vi "crio1_fpga.vi"() -> ()   [LabVIEW 2012]
uses:
  <vilib>/LabVIEW Targets/FPGA/cRIO/shared/nicrio_ModuleControls/nicrio_cRIO-9871_BaudRateEnum.ctl
  <vilib>/LabVIEW Targets/FPGA/cRIO/shared/nicrio_ModuleControls/nicrio_cRIO-9871_DataBitsEnum.ctl
  <vilib>/LabVIEW Targets/FPGA/cRIO/shared/nicrio_ModuleControls/nicrio_cRIO-9871_ParityEnum.ctl
  <vilib>/LabVIEW Targets/FPGA/cRIO/shared/nicrio_ModuleControls/nicrio_cRIO-9871_StopBitsEnum.ctl
  <vilib>/rvi/eio/common/nirviEmuTemplateMethod_errors.vi
  <vilib>/rvi/eio/common/nirviEmuTemplatePropertySet_noerrors.vi
  <vilib>/eio/EIONode/EIONode.xnode
  <vilib>/eio/EIOMethodNode/EIOMethodNode.xnode
  <vilib>/eio/EIOPropertyNode/EIOPropertyNode.xnode
  <vilib>/rvi/eio/common/nirviEmuTemplatePropertyGet_errors.vi
  <vilib>/rvi/eio/common/nirviEmuTemplatePropertyGet_noerrors.vi
  <vilib>/rvi/eio/common/nirviEmuTemplatePropertySet_errors.vi
panel:
  out "interlocked tripped":bool
  out "DI Gate Valves":bool[](array[boolean])
  in  "Mod8/CH2":bool
  in  "Mod8/CH4":bool
  in  "Mod8/CH3":bool
  out "DIO OUTPUT":bool[](array[boolean])
  out "Convectron 2":u8[](array[numeric])
  out "Ion gauge 1":u8[](array[numeric])
  out "Convectron 1":u8[](array[numeric])
  out "Ion gauge 2":u8[](array[numeric])
  in  "R45 Switch magnet Aperture":bool
  in  "R45 Switch magnet faraday cup":bool
  out "Analog input":fxp<+/-,26,5>[](array[numeric]) format="%.23g"
  in  "Analog Output":fxp<+/-,26,5>[](array[numeric])=[0.0, 0.0, 0.0, 0.0, 0.0, 0.0, 0.0, 0.0] format="%.23g"
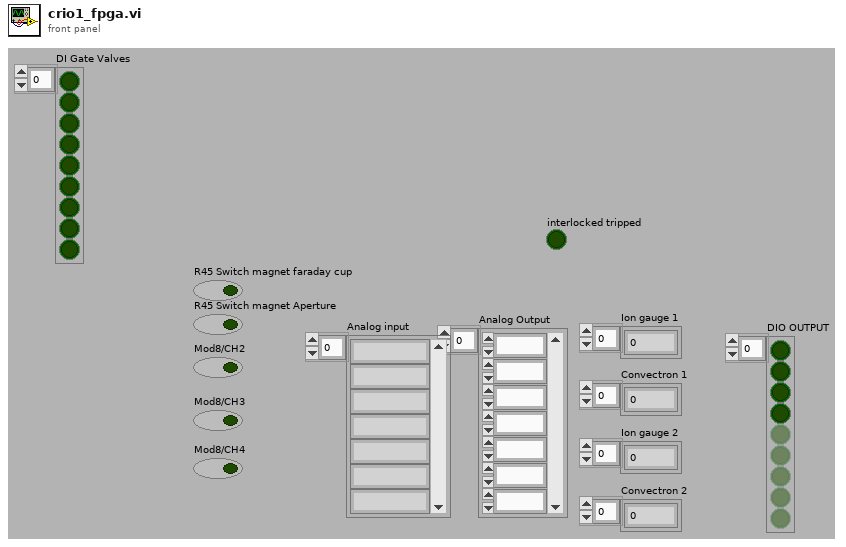
[diagram p1: front panel]
types:
  T1 = typedef "nicrio_cRIO-9871_StopBitsEnum.ctl" = enum8{"1", "1.5", "2"}
  T2 = typedef "nicrio_cRIO-9871_ParityEnum.ctl" = enum8{"None", "Odd", "Even", "Mark", "Space"}
  T3 = typedef "nicrio_cRIO-9871_DataBitsEnum.ctl" = enum8{"5", "6", "7", "8"}
  T4 = typedef "nicrio_cRIO-9871_BaudRateEnum.ctl" = enum16{"75 bps", "110 bps", "134 bps", "150 bps", "300 bps", "600 bps", "1200 bps", "1800 bps", "2400 bps", "4800 bps", "7200 bps", "9600 bps", "14.4 kbps", "19.2 kbps", "28.8 kbps", "38.4 kbps", "57.6 kbps", "115.2 kbps", "230.4 kbps", "460.8 kbps", "921.6 kbps"}
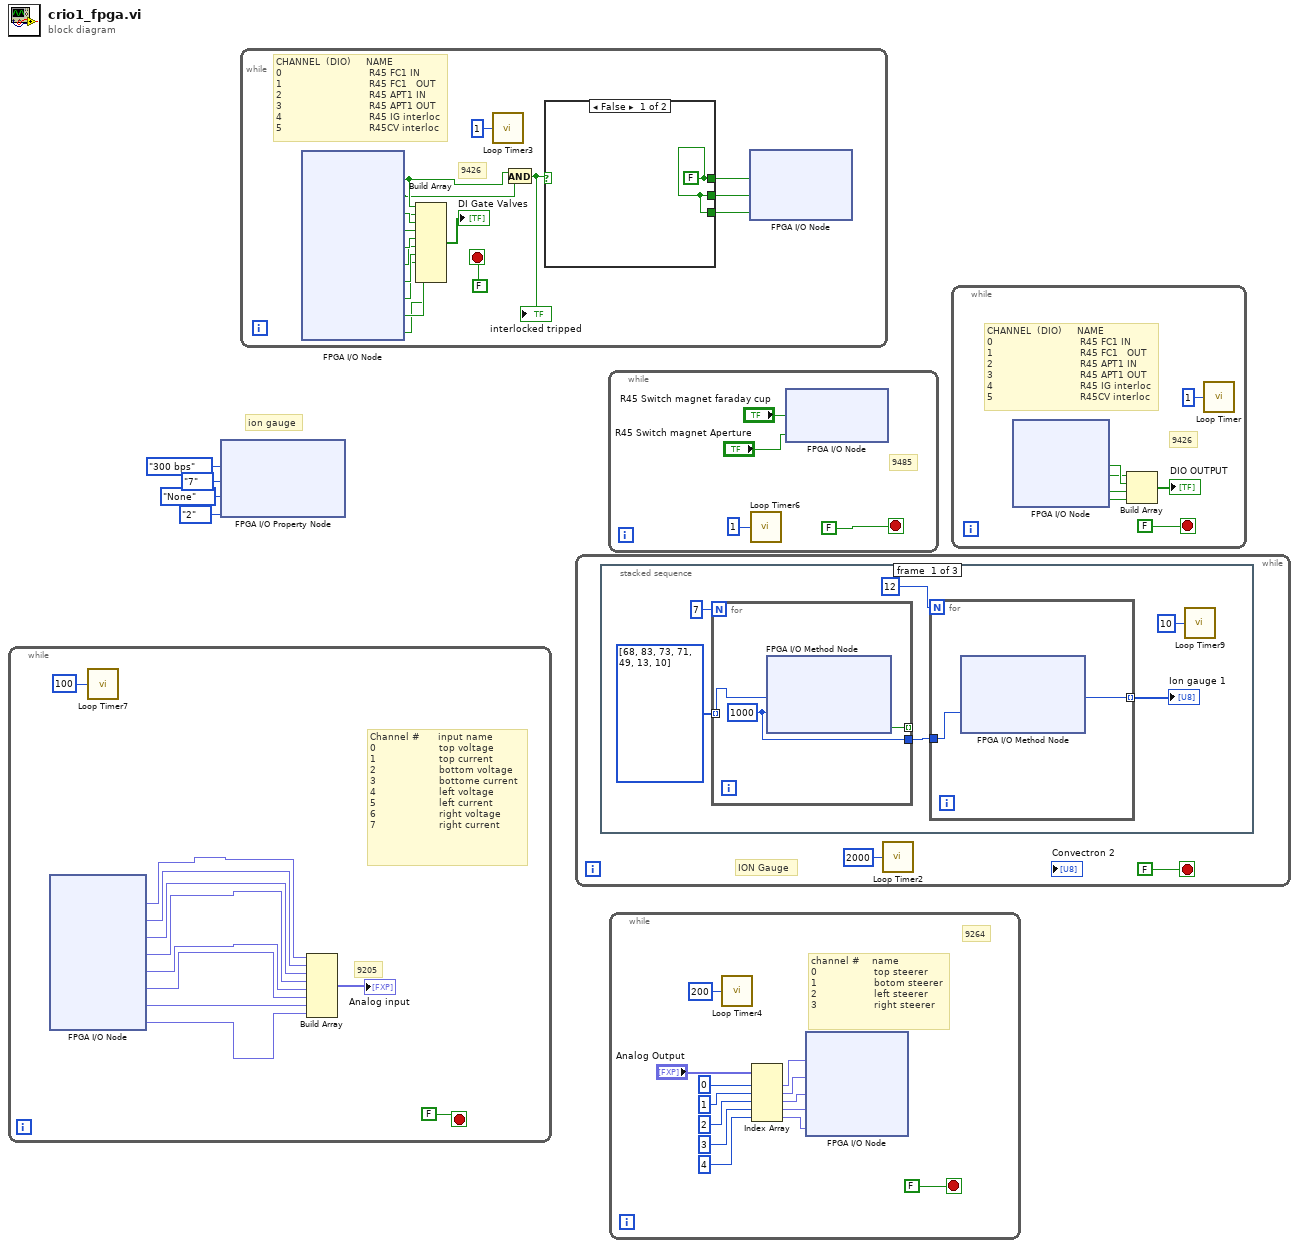
[diagram p0: block diagram]
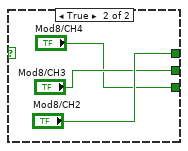
[diagram p2: hidden frame]
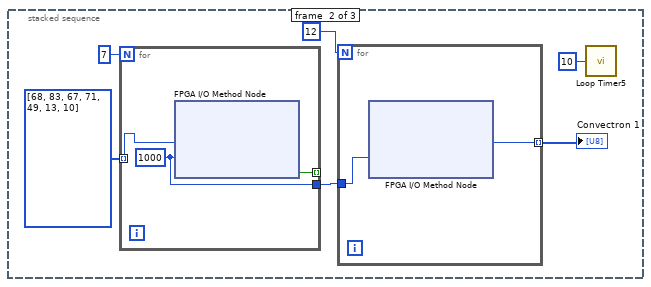
[diagram p3: hidden frame]
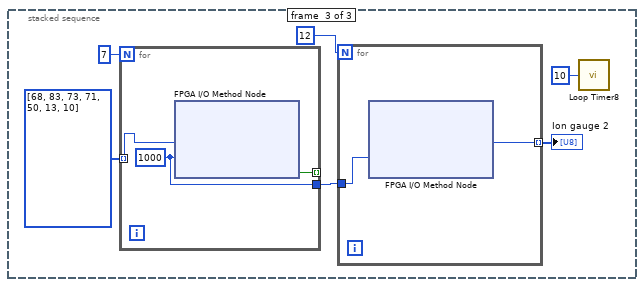
[diagram p4: hidden frame]
diagram:
  # "ion gauge"
  n1 = while {
    stop <- FALSE stop-if-true
    # "Channel #      input name\n0                     top voltage\n1                     top current\n2                     bottom voltage\n3                     bottome current\n4                     left voltage\n5                     left current\n6                     right voltage\n7                     right current"
    # "9205"
    n2 = xnode "FPGA I/O Node"() -> ("Mod1/AI0"=w13:fxp<+/-,26,5>, "Mod1/AI1"=w12:fxp<+/-,26,5>, "Mod1/AI2"=w11:fxp<+/-,26,5>, "Mod1/AI3"=w10:fxp<+/-,26,5>, "Mod1/AI4"=w9:fxp<+/-,26,5>, "Mod1/AI5"=w8:fxp<+/-,26,5>, "Mod1/AI6"=w7:fxp<+/-,26,5>, "Mod1/AI7"=w6:fxp<+/-,26,5>)  [unwired: 8 in, 8 out]
    n3 = call "Loop Timer7"("Count(mSec)"=u32 100 ("Count(Ticks)")) -> ()  [unwired: 1 out]
    n4 = Build Array(w13, w12, w11, w10, w9, w8, w7, w6) -> (→"Analog input":fxp<+/-,26,5>[])
  }
  n5 = xnode "FPGA I/O Property Node"("Baud Rate"=nicrio_cRIO-9871_BaudRateEnum."300 bps", "Data Bits"=nicrio_cRIO-9871_DataBitsEnum."7", "Parity"=nicrio_cRIO-9871_ParityEnum."None", "Stop Bits"=nicrio_cRIO-9871_StopBitsEnum."2") -> ()  [unwired: 1 in, 1 out]
  n6 = while {
    stop <- FALSE stop-if-true
    # "9426"
    # "CHANNEL  (DIO)     NAME\n0                             R45 FC1 IN\n1                             R45 FC1   OUT\n2                             R45 APT1 IN\n3                             R45 APT1 OUT\n4                             R45 IG interloc\n5                             R45CV interloc"
    n7 = xnode "FPGA I/O Node"() -> ("Mod7/DI4"=w21:bool, "Mod7/DI5"=w20:bool, "Mod7/DI6"=w29:bool, "Mod7/DI7"=w28:bool, "Mod7/DI8"=w27:bool, "Mod7/DI9"=w26:bool, "Mod7/DI10"=w19:bool, "Mod7/DI11"=w18:bool, "Mod7/DI12"=w17:bool, "Mod7/DI13"=w16:bool)  [unwired: 10 in, 10 out]
    n8 = Build Array(w21, w20, w29, w28, w27, w26, w19, w18, w17, w16) -> (→"DI Gate Valves":bool[])
    n9 = call "Loop Timer3"("Count(uSec)"=u32 1 ("Count(Ticks)")) -> ()  [unwired: 1 out]
    n10 = And(x=w21, y=w20) -> (x .and. y?=w22:bool)
    "interlocked tripped" <- w22
    n11 = case shown="False" w22 {
      tunnel: [w33 "Mod8/CH2"] -> w25
      tunnel: [w33 "Mod8/CH3"] -> w24
      tunnel: [w33 "Mod8/CH4"] -> w23
      frame False {
        w33 = FALSE ("Mod8/CH2")
      }
      frame True {
      }
    }
    n12 = xnode "FPGA I/O Node"("Mod8/CH2"=w25, "Mod8/CH3"=w24, "Mod8/CH4"=w23) -> ()  [unwired: 3 in, 3 out]
  }
  n13 = while {
    stop <- FALSE stop-if-true
    # "ION Gauge"
    n14 = stacked-sequence {
      frame #0 {
        n15 = for {
          N: 7 -> [_]
          tunnel: [w49] -> w44
          tunnel: [w48] -> _ mode=indexing
          tunnel: u8[] [68, 83, 73, 71, 49, 13, 10] ("unsigned byte array") -> [w47] mode=indexing
          w49 = 1000 ("Timeout (ms)")
          n16 = xnode "FPGA I/O Method Node"("Data"=w47, "Timeout (ms)"=w49) -> ("Timed Out"=w48:bool)  [unwired: 1 in, 1 out]
        }
        n17 = for {
          N: 12 -> [_]
          tunnel: w44 -> [w46]
          tunnel: [w45] -> w40 mode=indexing
          n18 = xnode "FPGA I/O Method Node"("Timeout (ms)"=w46) -> ("Data"=w45:u8)  [unwired: 1 in, 2 out]
        }
        "Ion gauge 1" <- w40
        n19 = call "Loop Timer9"("Count(mSec)"=u32 10 ("Count(Ticks)")) -> ()  [unwired: 1 out]
      }
      frame #1 {
        n20 = for {
          N: 7 -> [_]
          tunnel: [w60] -> w55
          tunnel: [w59] -> _ mode=indexing
          tunnel: u8[] [68, 83, 67, 71, 49, 13, 10] ("unsigned byte array") -> [w58] mode=indexing
          w60 = 1000 ("Timeout (ms)")
          n21 = xnode "FPGA I/O Method Node"("Data"=w58, "Timeout (ms)"=w60) -> ("Timed Out"=w59:bool)  [unwired: 1 in, 1 out]
        }
        n22 = for {
          N: 12 -> [_]
          tunnel: w55 -> [w57]
          tunnel: [w56] -> w51 mode=indexing
          n23 = xnode "FPGA I/O Method Node"("Timeout (ms)"=w57) -> ("Data"=w56:u8)  [unwired: 1 in, 2 out]
        }
        "Convectron 1" <- w51
        n24 = call "Loop Timer5"("Count(mSec)"=u32 10 ("Count(Ticks)")) -> ()  [unwired: 1 out]
      }
      frame #2 {
        n25 = for {
          N: 7 -> [_]
          tunnel: [w71] -> w66
          tunnel: [w70] -> _ mode=indexing
          tunnel: u8[] [68, 83, 73, 71, 50, 13, 10] ("unsigned byte array") -> [w69] mode=indexing
          w71 = 1000 ("Timeout (ms)")
          n26 = xnode "FPGA I/O Method Node"("Data"=w69, "Timeout (ms)"=w71) -> ("Timed Out"=w70:bool)  [unwired: 1 in, 1 out]
        }
        n27 = for {
          N: 12 -> [_]
          tunnel: w66 -> [w68]
          tunnel: [w67] -> w62 mode=indexing
          n28 = xnode "FPGA I/O Method Node"("Timeout (ms)"=w68) -> ("Data"=w67:u8)  [unwired: 1 in, 2 out]
        }
        "Ion gauge 2" <- w62
        n29 = call "Loop Timer8"("Count(mSec)"=u32 10 ("Count(Ticks)")) -> ()  [unwired: 1 out]
      }
    }
    n30 = call "Loop Timer2"("Count(mSec)"=u32 2000 ("Count(Ticks)")) -> ()  [unwired: 1 out]
  }
  n31 = while {
    stop <- FALSE stop-if-true
    # "9485"
    n32 = call "Loop Timer6"("Count(mSec)"=u32 1 ("Count(Ticks)")) -> ()  [unwired: 1 out]
    n33 = xnode "FPGA I/O Node"("Mod8/CH0"="R45 Switch magnet faraday cup", "Mod8/CH1"="R45 Switch magnet Aperture") -> ()  [unwired: 2 in, 2 out]
  }
  n34 = while {
    stop <- FALSE stop-if-true
    # "9264"
    # "channel #    name\n0                   top steerer\n1                   botom steerer\n2                   left steerer\n3                   right steerer"
    n35 = call "Loop Timer4"("Count(mSec)"=u32 200 ("Count(Ticks)")) -> ()  [unwired: 1 out]
    n36 = Index Array(array="Analog Output", index #1=0 ("index"), index #2=1 ("index"), index #3=2 ("index"), index #4=3 ("index"), index #5=4 ("index")) -> (element #1=w81:fxp<+/-,26,5>, element #2=w80:fxp<+/-,26,5>, element #3=w79:fxp<+/-,26,5>, element #4=w78:fxp<+/-,26,5>, element #5=w76:fxp<+/-,26,5>)
    n37 = xnode "FPGA I/O Node"("Mod2/AO0"=w81, "Mod2/AO1"=w80, "Mod2/AO2"=w79, "Mod2/AO3"=w78, "Mod2/AO4"=w76) -> ()  [unwired: 5 in, 5 out]
  }
  n38 = while {
    stop <- FALSE stop-if-true
    # "9426"
    # "CHANNEL  (DIO)     NAME\n0                             R45 FC1 IN\n1                             R45 FC1   OUT\n2                             R45 APT1 IN\n3                             R45 APT1 OUT\n4                             R45 IG interloc\n5                             R45CV interloc"
    n39 = xnode "FPGA I/O Node"() -> ("Mod7/DI0"=w89:bool, "Mod7/DI1"=w90:bool, "Mod7/DI2"=w91:bool, "Mod7/DI3"=w92:bool)  [unwired: 4 in, 4 out]
    n40 = Build Array(w89, w90, w91, w92) -> (→"DIO OUTPUT":bool[])
    n41 = call "Loop Timer"("Count(mSec)"=u32 1 ("Count(Ticks)")) -> ()  [unwired: 1 out]
  }
